vi "Autonomous Independent.vi"   [LabVIEW 2015]
doc: "This VI is called when autonomous begins, and will automatically be terminated when autonomous ends. You can carry out timed or sensor driven robot movement independently without needing to return to the caller."
uses:
  <vilib>/Rock Robotics/WPI/Solenoid/WPI_SolenoidValue.ctl
  <vilib>/Rock Robotics/WPI/Utilities/WPI_GetSetVariantRefNum.vi
  <vilib>/Rock Robotics/Network Tables/NT Read String.vi
  Robot Global Data.vi
  <vilib>/Rock Robotics/Network Tables/NT Write Number.vi
  <vilib>/Rock Robotics/WPI/Solenoid/Deprecated/WPI_SolenoidGetBool.vi
  <vilib>/Rock Robotics/WPI/Solenoid/WPI_SolenoidSetEnum.vi
  <vilib>/Rock Robotics/WPI/RobotDrive/WPI_RobotDriveArcadeDrive_Standard(NoSaturation).vi
  <vilib>/Rock Robotics/Network Tables/NT Write Numeric Array.vi
panel:
  # "Be sure to right-click and choose Data Operations>>Make Current Value default if you want to save the array values with the VI"
types:
  T1 = typedef "WPI_JoystickDevRef.ctl" = cluster{"Device":T2}
  T2 = typedef "WPI_JoystickDeviceEnum.ctl" = enum16{"USB 0", "USB 1", "USB 2", "USB 3", "USB 4", "USB 5"}
  T3 = typedef "WPI_SolenoidValue.ctl" = enum16{"Off", "On", "Forward", "Reverse"}
  T4 = typedef "WPI_RobotDriveDevRef.ctl" = cluster{"DevStatus":errorcluster, "Motors[]":T5[], "Square Inputs":bool, "Max Output":dbl}
  T5 = typedef "WPI_MotorControlDeviceRef.ctl" = cluster{"DeviceStatus":errorcluster, "Type":T6, "PWM":cluster{"PWM Channel":T7, "DeadBand":T8}, "CAN":cluster{"Device Number":u8, "Control Mode":T9, "Semaphore":T10, "Max Vout":dbl, "TalonSRX Control Mode":T11}, "Invert":bool}
  T6 = typedef "WPI_MotorControlType.ctl" = enum16{"PWM", "CAN", "CANTalonSRX"}
  T7 = typedef "FPGA_DIOPWMChannel.ctl" = enum8{"PWM 0", "PWM 1", "PWM 2", "PWM 3", "PWM 4", "PWM 5", "PWM 6", "PWM 7", "PWM 8", "PWM 9", "PWM MXP 0", "PWM MXP 1", "PWM MXP 2", "PWM MXP 3", "PWM MXP 4", "PWM MXP 5", "PWM MXP 6", "PWM MXP 7", "PWM MXP 8", "PWM MXP 9", "Invalid"}
  T8 = typedef "WPI_PWMDeadband.ctl" = cluster{"Name":string, "maxPositivePwm":i32, "minPositivePwm":i32, "centerPwm":i32, "maxNegativePwm":i32, "minNegativePwm":i32, "angularRange":u16}
  T9 = typedef "WPI_CANJaguar_ControlMode.ctl" = enum8{"Percent VBus", "Current", "Speed", "Position", "Voltage"}
  T10 = typedef "Semaphore RefNum" = refnum<k1>
  T11 = typedef "WPI_CANTalonSRX_APIControlMode.ctl" = enum8{"Percent VBus", "Speed", "Position", "Slave", "Unchanged / Invalid", "Voltage Compensation", "Current", "Motion Profile"}
  T12 = typedef "WPI_GyroDevRef.ctl" = cluster{"DevStatus":errorcluster, "Analog Channel":T13, "Offset":dbl, "Gain (VoltsPerDegree/Second)":dbl, "Gyro Type":enum16{"Analog", "XRS450"}, "Handle":i32, "SPI Bus":T14, "Device Found":bool, "Sample Rate":dbl, "Calibrate On Open":bool}
  T13 = typedef "FPGA_AIChannel.ctl" = enum8{"AI 0", "AI 1", "AI 2", "AI 3", "AI MXP 0", "AI MXP 1", "AI MXP 2", "AI MXP 3", "Invalid"}
  T14 = typedef "spi_bus.ctl" = enum16{"SPI On-Board, CS0", "SPI On-Board, CS1", "SPI On-Board, CS2", "SPI On-Board, CS3", "SPI MXP", "Invalid"}
  T15 = typedef "WPI_PotentiometerDevRef.ctl" = cluster{"DevStatus":errorcluster, "Analog Channel":T13, "Invert Output":bool}
  T16 = typedef "WPI_SolenoidDevRef.ctl" = cluster{"DevStatus":errorcluster, "Pneumatics Control Module":u8, "Forward Solenoid Channel":T17, "Reverse Solenoid Channel":T17}
  T17 = typedef "WPI_SolenoidChannel.ctl" = enum8{"Solenoid 0", "Solenoid 1", "Solenoid 2", "Solenoid 3", "Solenoid 4", "Solenoid 5", "Solenoid 6", "Solenoid 7", "Invalid"}
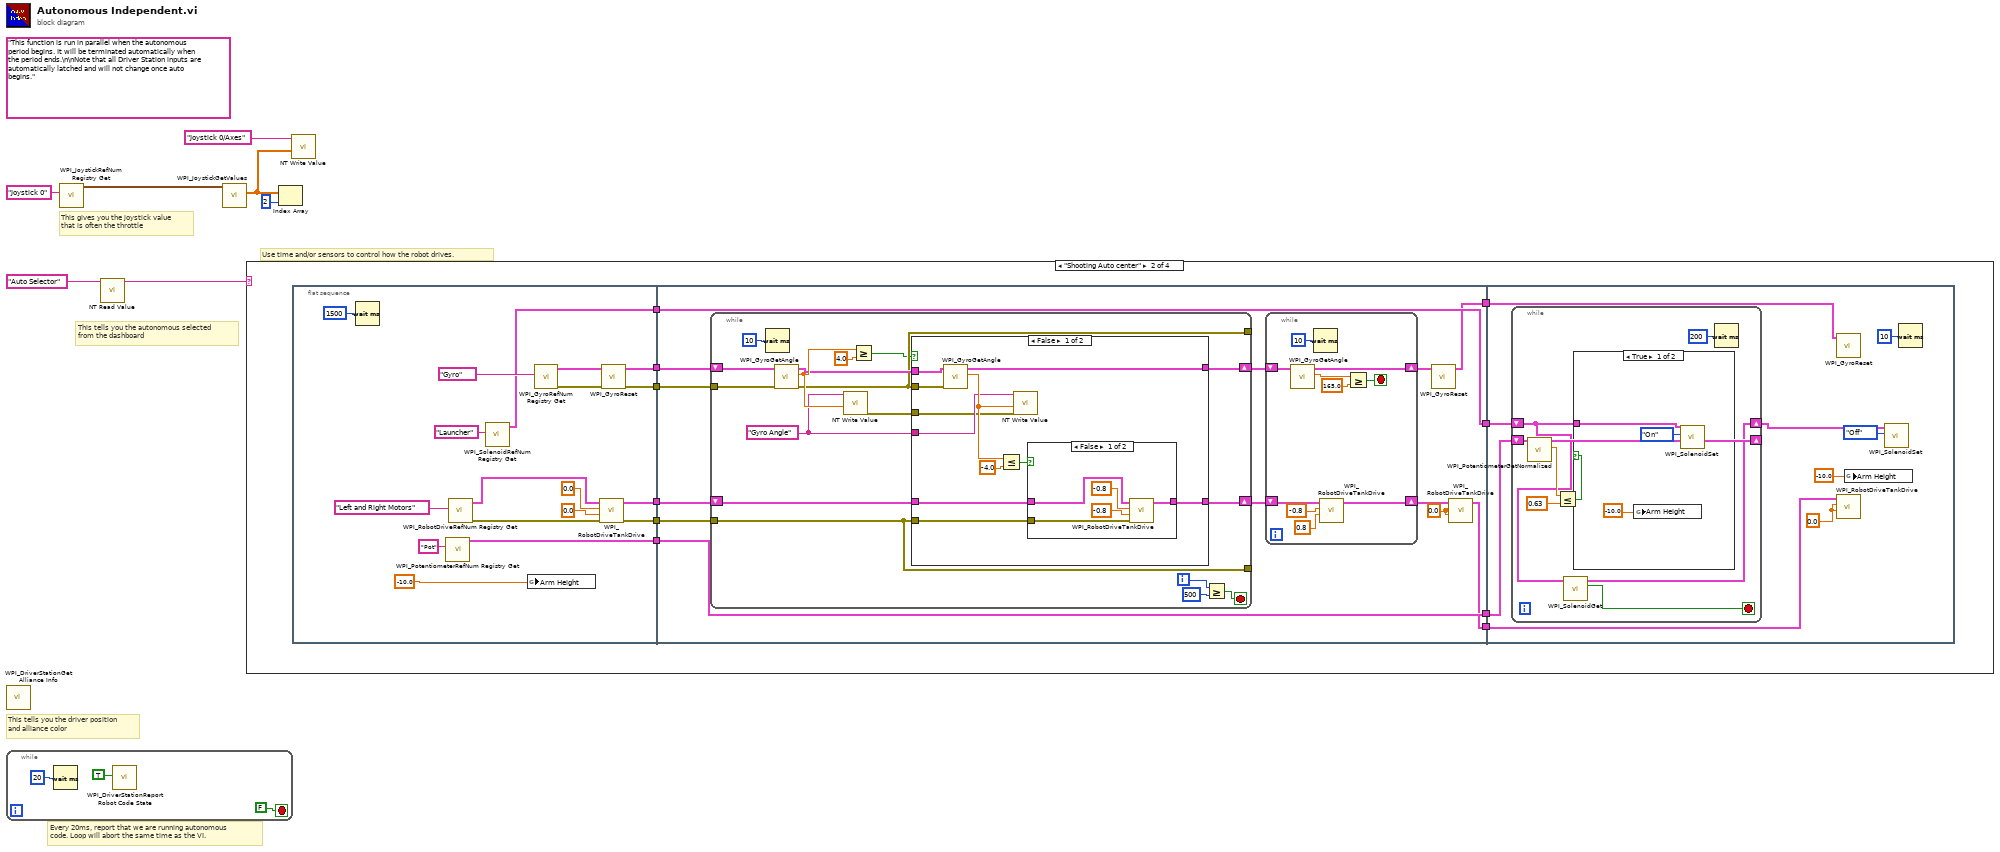
[diagram p0: block diagram]
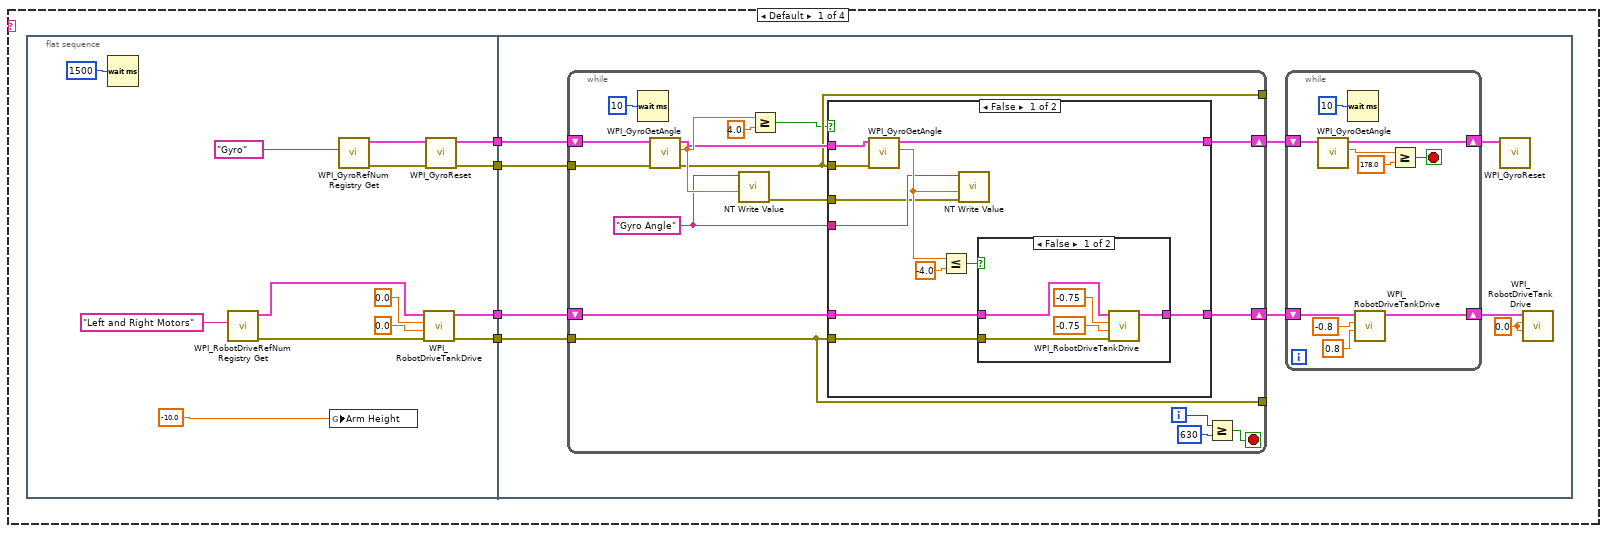
[diagram p2: hidden frame]
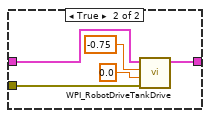
[diagram p3: hidden frame]
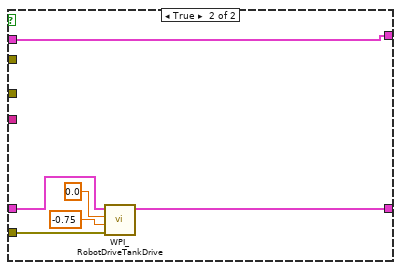
[diagram p4: hidden frame]
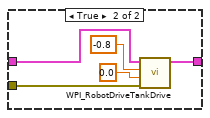
[diagram p5: hidden frame]
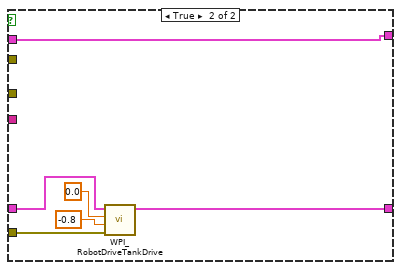
[diagram p6: hidden frame]
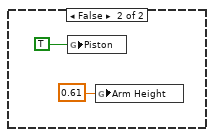
[diagram p7: hidden frame]
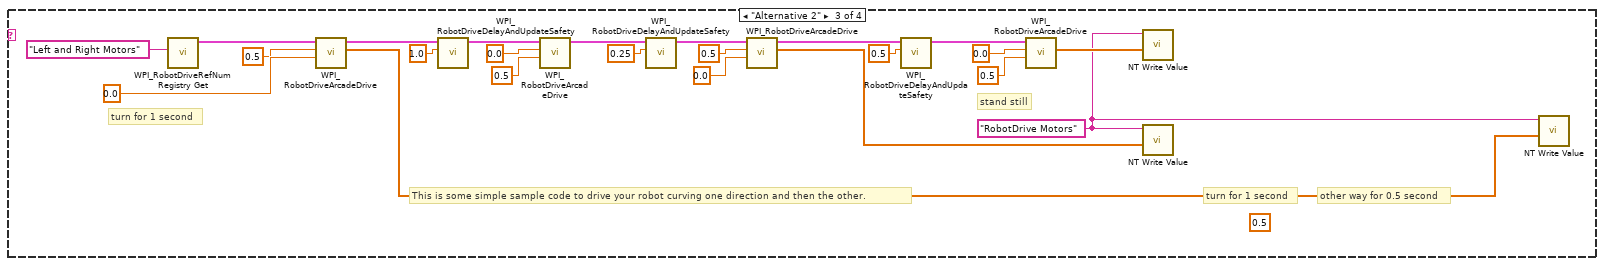
[diagram p8: hidden frame]
diagram:
  (unwired) "This function is run in parallel when the autonomous period begins. It will be terminated automatically when the period ends.\n\nNote that all Driver Station inputs are automatically latched and will not change once auto begins."
  # "This tells you the autonomous selected\nfrom the dashboard"
  # "Every 20ms, report that we are running autonomous\ncode. Loop will abort the same time as the VI."
  # "This gives you the joystick value\nthat is often the throttle"
  # "Use time and/or sensors to control how the robot drives."
  # "This tells you the driver position\nand alliance color"
  n1 = call <vilib>:"WPI_DriverStationGet Alliance Info.vi"() -> ()  [unwired: 12 out]
  n2 = while {
    stop <- FALSE stop-if-true
    n3 = Wait (ms)(milliseconds to wait=u32 20) -> ()  [unwired: 1 out]
    n4 = call <vilib>:"WPI_DriverStationReport Robot Code State.vi"("Autonomous"=TRUE) -> ()  [unwired: 10 in, 1 out]
  }
  n5 = call <vilib>:"WPI_JoystickRefNum Registry Get.vi"("refnum name"="Joystick 0") -> ("JoystickDevRef"=w6:T1)  [unwired: 1 in, 9 out]
  n6 = call-poly <vilib>:"NT Read Value.vi"("Name"="Auto Selector") -> ("String"=w3:string)  [unwired: 9 in, 1 out]
  n7 = call <vilib>:"WPI_JoystickGetValues.vi"("JoystickDevRef"=w6) -> ("Axes"=w2:dbl[])  [unwired: 6 in, 4 out]
  n8 = case shown="\"Shooting Auto center\"" w3 {
    frame Default {
      n9 = flat-sequence {
        tunnel: [w21] -> w14
        tunnel: [w20] -> w13
        tunnel: [w19] -> w12
        tunnel: [w18] -> w11
        tunnel: w14 -> [w37]
        tunnel: w13 -> [w36]
        tunnel: w12 -> [w35]
        tunnel: w11 -> [w34]
        frame #0 {
          n10 = Wait (ms)(milliseconds to wait=u32 1500) -> ()  [unwired: 1 out]
          n11 = call <vilib>:"WPI_RobotDriveRefNum Registry Get.vi"("refnum name"="Left and Right Motors") -> ("error out"=w24:errorcluster, "RobotDriveDevRef"=w25:T4)  [unwired: 9 in]
          n12 = global write "Robot Global Data.vi" "Arm Height"(-10.0) -> ()
          n13 = call <vilib>:"WPI_GyroRefNum Registry Get.vi"("refnum name"="Gyro") -> ("error out"=w27:errorcluster, "GyroDevRef"=w28:T12)  [unwired: 9 in]
          n14 = call <vilib>:"WPI_RobotDriveTankDrive.vi"("error in (no error)"=w24, "Right axis value"=0.0, "Left axis value"=0.0 ("Delay (s)"), "RobotDriveDevRef"=w25) -> ("error out"=w18:errorcluster, "RobotDriveDevRef"=w19:T4)  [unwired: 5 in, 1 out]
          n15 = call <vilib>:"WPI_GyroReset.vi"("error in"=w27, "GyroDevRef"=w28) -> ("error out"=w20:errorcluster, "GyroDevRef"=w21:T12)  [unwired: 8 in]
        }
        frame #1 {
          w30 = 0.0 ("Left axis value")
          n16 = while {
            tunnel: w36 -> [w61]
            tunnel: w34 -> [w56]
            tunnel: [w57] -> _
            tunnel: [w56] -> _
            shift-right: [w49] -> w33
            shift-left: w35 -> [w55]
            shift-right: [w48] -> w32
            shift-left: w37 -> [w64]
            i -> [w50]
            stop <- w62 stop-if-true
            w54 = "Gyro Angle" ("Name")
            n17 = Wait (ms)(milliseconds to wait=10) -> ()  [unwired: 1 out]
            n18 = call <vilib>:"WPI_GyroGetAngle.vi"("error in"=w61, "GyroDevRef"=w64) -> ("error out"=w57:errorcluster, "Angle"=w59:dbl, "GyroDevRef"=w58:T12)  [unwired: 5 in, 2 out]
            n19 = call-poly <vilib>:"NT Write Value.vi"("Numeric"=w59, "Name"=w54) -> ("error out"=w53:errorcluster)  [unwired: 9 in]
            n20 = Greater Or Equal?(x=w59, y=4.0) -> (x >= y?=w52:bool)
            n21 = case shown="False" w52 {
              tunnel: w56 -> [w71 w88]
              tunnel: w55 -> [w72 w89]
              tunnel: w58 -> [w75 w86]
              tunnel: w57 -> [w74 _]
              tunnel: w54 -> [w69 _]
              tunnel: w53 -> [w68 _]
              tunnel: [w66 w87] -> w49
              tunnel: [w65 w86] -> w48
              frame False {
                n22 = call <vilib>:"WPI_GyroGetAngle.vi"("error in"=w74, "GyroDevRef"=w75) -> ("Angle"=w70:dbl, "GyroDevRef"=w65:T12)  [unwired: 5 in, 3 out]
                n23 = Less Or Equal?(x=w70, y=-4.0) -> (x <= y?=w67:bool)
                n24 = call-poly <vilib>:"NT Write Value.vi"("error in"=w68, "Numeric"=w70, "Name"=w69) -> ()  [unwired: 8 in, 1 out]
                n25 = case shown="False" w67 {
                  tunnel: w72 -> [w80 w85]
                  tunnel: w71 -> [w79 w84]
                  tunnel: [w76 w81] -> w66
                  frame False {
                    n26 = call <vilib>:"WPI_RobotDriveTankDrive.vi"("error in (no error)"=w79, "Right axis value"=-0.75, "Left axis value"=-0.75, "RobotDriveDevRef"=w80) -> ("RobotDriveDevRef"=w76:T4)  [unwired: 5 in, 2 out]
                  }
                  frame True {
                    n27 = call <vilib>:"WPI_RobotDriveTankDrive.vi"("error in (no error)"=w84, "Right axis value"=0.0, "Left axis value"=-0.75, "RobotDriveDevRef"=w85) -> ("RobotDriveDevRef"=w81:T4)  [unwired: 5 in, 2 out]
                  }
                }
              }
              frame True {
                n28 = call <vilib>:"WPI_RobotDriveTankDrive.vi"("error in (no error)"=w88, "Right axis value"=-0.75, "Left axis value"=0.0, "RobotDriveDevRef"=w89) -> ("RobotDriveDevRef"=w87:T4)  [unwired: 5 in, 2 out]
              }
            }
            n29 = Greater Or Equal?(x=w50, y=u32 630) -> (x >= y?=w62:bool)
          }
          n30 = while {
            shift-right: [w39] -> w31
            shift-left: w32 -> [w46]
            shift-right: [w40] -> w29
            shift-left: w33 -> [w47]
            stop <- w41 stop-if-true
            n31 = call <vilib>:"WPI_GyroGetAngle.vi"("GyroDevRef"=w46) -> ("Angle"=w43:dbl, "GyroDevRef"=w39:T12)  [unwired: 6 in, 3 out]
            n32 = Wait (ms)(milliseconds to wait=u32 10) -> ()  [unwired: 1 out]
            n33 = call <vilib>:"WPI_RobotDriveTankDrive.vi"("Right axis value"=0.8, "Left axis value"=-0.8, "RobotDriveDevRef"=w47) -> ("RobotDriveDevRef"=w40:T4)  [unwired: 6 in, 2 out]
            n34 = Greater Or Equal?(x=w43, y=178.0) -> (x >= y?=w41:bool)
          }
          n35 = call <vilib>:"WPI_GyroReset.vi"("GyroDevRef"=w31) -> ()  [unwired: 9 in, 2 out]
          n36 = call <vilib>:"WPI_RobotDriveTankDrive.vi"("Right axis value"=w30, "Left axis value"=w30, "RobotDriveDevRef"=w29) -> ()  [unwired: 6 in, 3 out]
        }
      }
    }
    frame "Shooting Auto center" {
      n37 = flat-sequence {
        tunnel: [w112] -> w101
        tunnel: [w111] -> w100
        tunnel: [w110] -> w99
        tunnel: [w109] -> w98
        tunnel: [w103] -> w96
        tunnel: [w102] -> w94
        tunnel: w101 -> [w132]
        tunnel: w100 -> [w131]
        tunnel: w99 -> [w130]
        tunnel: w98 -> [w129]
        tunnel: [w123] -> w97
        tunnel: w96 -> [w123]
        tunnel: [w122] -> w95
        tunnel: w94 -> [w122]
        tunnel: [w121] -> w93
        tunnel: [w120] -> w92
        tunnel: w97 -> [w195]
        tunnel: w95 -> [w194]
        tunnel: w93 -> [w191]
        tunnel: w92 -> [w190]
        frame #0 {
          n38 = Wait (ms)(milliseconds to wait=u32 1500) -> ()  [unwired: 1 out]
          n39 = call <vilib>:"WPI_PotentiometerRefNum Registry Get.vi"("refnum name"="Pot") -> ("PotDevRef"=w103:T15)  [unwired: 9 in, 1 out]
          n40 = call <vilib>:"WPI_RobotDriveRefNum Registry Get.vi"("refnum name"="Left and Right Motors") -> ("error out"=w115:errorcluster, "RobotDriveDevRef"=w116:T4)  [unwired: 9 in]
          n41 = call <vilib>:"WPI_SolenoidRefNum Registry Get.vi"("refnum name"="Launcher") -> ("SolenoidDevRef"=w102:T16)  [unwired: 9 in, 1 out]
          n42 = global write "Robot Global Data.vi" "Arm Height"(-10.0) -> ()
          n43 = call <vilib>:"WPI_GyroRefNum Registry Get.vi"("refnum name"="Gyro") -> ("error out"=w118:errorcluster, "GyroDevRef"=w119:T12)  [unwired: 9 in]
          n44 = call <vilib>:"WPI_RobotDriveTankDrive.vi"("error in (no error)"=w115, "Right axis value"=0.0, "Left axis value"=0.0 ("Delay (s)"), "RobotDriveDevRef"=w116) -> ("error out"=w109:errorcluster, "RobotDriveDevRef"=w110:T4)  [unwired: 5 in, 1 out]
          n45 = call <vilib>:"WPI_GyroReset.vi"("error in"=w118, "GyroDevRef"=w119) -> ("error out"=w111:errorcluster, "GyroDevRef"=w112:T12)  [unwired: 8 in]
        }
        frame #1 {
          w125 = 0.0 ("Left axis value")
          n46 = while {
            tunnel: w131 -> [w156]
            tunnel: w129 -> [w151]
            tunnel: [w152] -> _
            tunnel: [w151] -> _
            shift-right: [w144] -> w128
            shift-left: w130 -> [w150]
            shift-right: [w143] -> w127
            shift-left: w132 -> [w159]
            i -> [w145]
            stop <- w157 stop-if-true
            w149 = "Gyro Angle" ("Name")
            n47 = Wait (ms)(milliseconds to wait=10) -> ()  [unwired: 1 out]
            n48 = call <vilib>:"WPI_GyroGetAngle.vi"("error in"=w156, "GyroDevRef"=w159) -> ("error out"=w152:errorcluster, "Angle"=w154:dbl, "GyroDevRef"=w153:T12)  [unwired: 5 in, 2 out]
            n49 = call-poly <vilib>:"NT Write Value.vi"("Numeric"=w154, "Name"=w149) -> ("error out"=w148:errorcluster)  [unwired: 9 in]
            n50 = Greater Or Equal?(x=w154, y=4.0) -> (x >= y?=w147:bool)
            n51 = case shown="False" w147 {
              tunnel: w151 -> [w166 w183]
              tunnel: w150 -> [w167 w184]
              tunnel: w153 -> [w170 w181]
              tunnel: w152 -> [w169 _]
              tunnel: w149 -> [w164 _]
              tunnel: w148 -> [w163 _]
              tunnel: [w161 w182] -> w144
              tunnel: [w160 w181] -> w143
              frame False {
                n52 = call <vilib>:"WPI_GyroGetAngle.vi"("error in"=w169, "GyroDevRef"=w170) -> ("Angle"=w165:dbl, "GyroDevRef"=w160:T12)  [unwired: 5 in, 3 out]
                n53 = Less Or Equal?(x=w165, y=-4.0) -> (x <= y?=w162:bool)
                n54 = call-poly <vilib>:"NT Write Value.vi"("error in"=w163, "Numeric"=w165, "Name"=w164) -> ()  [unwired: 8 in, 1 out]
                n55 = case shown="False" w162 {
                  tunnel: w167 -> [w175 w180]
                  tunnel: w166 -> [w174 w179]
                  tunnel: [w171 w176] -> w161
                  frame False {
                    n56 = call <vilib>:"WPI_RobotDriveTankDrive.vi"("error in (no error)"=w174, "Right axis value"=-0.8, "Left axis value"=-0.8, "RobotDriveDevRef"=w175) -> ("RobotDriveDevRef"=w171:T4)  [unwired: 5 in, 2 out]
                  }
                  frame True {
                    n57 = call <vilib>:"WPI_RobotDriveTankDrive.vi"("error in (no error)"=w179, "Right axis value"=0.0, "Left axis value"=-0.8, "RobotDriveDevRef"=w180) -> ("RobotDriveDevRef"=w176:T4)  [unwired: 5 in, 2 out]
                  }
                }
              }
              frame True {
                n58 = call <vilib>:"WPI_RobotDriveTankDrive.vi"("error in (no error)"=w183, "Right axis value"=-0.8, "Left axis value"=0.0, "RobotDriveDevRef"=w184) -> ("RobotDriveDevRef"=w182:T4)  [unwired: 5 in, 2 out]
              }
            }
            n59 = Greater Or Equal?(x=w145, y=u32 500) -> (x >= y?=w157:bool)
          }
          n60 = while {
            shift-right: [w134] -> w126
            shift-left: w127 -> [w141]
            shift-right: [w135] -> w124
            shift-left: w128 -> [w142]
            stop <- w136 stop-if-true
            n61 = call <vilib>:"WPI_GyroGetAngle.vi"("GyroDevRef"=w141) -> ("Angle"=w138:dbl, "GyroDevRef"=w134:T12)  [unwired: 6 in, 3 out]
            n62 = Wait (ms)(milliseconds to wait=u32 10) -> ()  [unwired: 1 out]
            n63 = call <vilib>:"WPI_RobotDriveTankDrive.vi"("Right axis value"=0.8, "Left axis value"=-0.8, "RobotDriveDevRef"=w142) -> ("RobotDriveDevRef"=w135:T4)  [unwired: 6 in, 2 out]
            n64 = Greater Or Equal?(x=w138, y=165.0) -> (x >= y?=w136:bool)
          }
          n65 = call <vilib>:"WPI_GyroReset.vi"("GyroDevRef"=w126) -> ("GyroDevRef"=w121:T12)  [unwired: 9 in, 1 out]
          n66 = call <vilib>:"WPI_RobotDriveTankDrive.vi"("Right axis value"=w125, "Left axis value"=w125, "RobotDriveDevRef"=w124) -> ("RobotDriveDevRef"=w120:T4)  [unwired: 6 in, 2 out]
        }
        frame #2 {
          w189 = 0.0
          n67 = while {
            shift-right: [w200] -> _
            shift-left: w195 -> [w201]
            shift-right: [w198] -> w193
            shift-left: w194 -> [w199]
            stop <- w197 stop-if-true
            n68 = call <vilib>:"WPI_PotentiometerGetNormalized.vi"("PotDevRef"=w201) -> ("Normalized Value"=w204:dbl, "PotDevRef"=w200:T15)  [unwired: 8 in, 1 out]
            n69 = Less Or Equal?(x=w204, y=0.63) -> (x <= y?=w202:bool)
            n70 = call-poly <vilib>:"WPI_SolenoidGet.vi"("SolenoidDevRef"=w199) -> ("Value"=w197:bool, "SolenoidDevRef"=w198:T16)  [unwired: 8 in, 1 out]
            n71 = case shown="True" w202 {
              tunnel: w199 -> [w205 _]
              frame True {
                n72 = global write "Robot Global Data.vi" "Arm Height"(-10.0) -> ()
                n73 = call-poly <vilib>:"WPI_SolenoidSet.vi"("Value"=WPI_SolenoidValue."On", "SolenoidDevRef"=w205) -> ()  [unwired: 8 in, 2 out]
              }
              frame False {
                n74 = global write "Robot Global Data.vi" "Piston"(TRUE ("Piston")) -> ()
                n75 = global write "Robot Global Data.vi" "Arm Height"(0.61) -> ()
              }
            }
            n76 = Wait (ms)(milliseconds to wait=u32 200) -> ()  [unwired: 1 out]
          }
          n77 = call <vilib>:"WPI_GyroReset.vi"("GyroDevRef"=w191) -> ()  [unwired: 9 in, 2 out]
          n78 = call <vilib>:"WPI_RobotDriveTankDrive.vi"("Right axis value"=w189, "Left axis value"=w189, "RobotDriveDevRef"=w190) -> ()  [unwired: 6 in, 3 out]
          n79 = global write "Robot Global Data.vi" "Arm Height"(-10.0) -> ()
          n80 = call-poly <vilib>:"WPI_SolenoidSet.vi"("Value"=WPI_SolenoidValue."Off", "SolenoidDevRef"=w193) -> ()  [unwired: 8 in, 2 out]
          n81 = Wait (ms)(milliseconds to wait=u32 10) -> ()  [unwired: 1 out]
        }
      }
    }
    frame "Alternative 2" {
      (unwired) 0.5 ("X axis value")
      w220 = "RobotDrive Motors" ("Name")
      # "turn for 1 second"
      # "This is some simple sample code to drive your robot curving one direction and then the other."
      # "stand still"
      # "other way for 0.5 second"
      # "turn for 1 second"
      n82 = call <vilib>:"WPI_RobotDriveRefNum Registry Get.vi"("refnum name"="Left and Right Motors") -> ("RobotDriveDevRef"=w232:T4)  [unwired: 1 in, 9 out]
      n83 = call-poly <vilib>:"WPI_RobotDriveArcadeDrive.vi"("Y axis value"=0.0 ("X axis value"), "X axis value"=0.5, "RobotDriveDevRef"=w232) -> ("Motor Values"=w219:dbl[], "RobotDriveDevRef"=w226:T4)  [unwired: 1 in, 6 out]
      n84 = call <vilib>:"WPI_RobotDriveDelayAndUpdateSafety.vi"("Delay (s)"=1.0, "RobotDriveDevRef"=w226) -> ("RobotDriveDevRef 2"=w217:T4)  [unwired: 8 in, 1 out]
      n85 = call-poly <vilib>:"WPI_RobotDriveArcadeDrive.vi"("Y axis value"=0.5 ("X axis value"), "X axis value"=0.0, "RobotDriveDevRef"=w217) -> ("RobotDriveDevRef"=w214:T4)  [unwired: 1 in, 7 out]
      n86 = call <vilib>:"WPI_RobotDriveDelayAndUpdateSafety.vi"("Delay (s)"=0.25, "RobotDriveDevRef"=w214) -> ("RobotDriveDevRef 2"=w213:T4)  [unwired: 8 in, 1 out]
      n87 = call-poly <vilib>:"WPI_RobotDriveArcadeDrive.vi"("Y axis value"=0.0 ("X axis value"), "X axis value"=0.5, "RobotDriveDevRef"=w213) -> ("Motor Values"=w221:dbl[], "RobotDriveDevRef"=w227:T4)  [unwired: 1 in, 6 out]
      n88 = call <vilib>:"WPI_RobotDriveDelayAndUpdateSafety.vi"("Delay (s)"=0.5, "RobotDriveDevRef"=w227) -> ("RobotDriveDevRef 2"=w228:T4)  [unwired: 8 in, 1 out]
      n89 = call-poly <vilib>:"WPI_RobotDriveArcadeDrive.vi"("Y axis value"=0.5 ("X axis value"), "X axis value"=0.0, "RobotDriveDevRef"=w228) -> ("Motor Values"=w222:dbl[])  [unwired: 1 in, 7 out]
      n90 = call-poly <vilib>:"NT Write Value.vi"("Numeric Array"=w222, "Name"=w220) -> ()  [unwired: 9 in, 1 out]
      n91 = call-poly <vilib>:"NT Write Value.vi"("Numeric Array"=w221, "Name"=w220) -> ()  [unwired: 9 in, 1 out]
      n92 = call-poly <vilib>:"NT Write Value.vi"("Numeric Array"=w219, "Name"=w220) -> ()  [unwired: 9 in, 1 out]
    }
    frame "Your Turn" {
    }
  }
  n93 = Index Array(array=w2, index=2) -> ()  [unwired: 1 out]
  n94 = call-poly <vilib>:"NT Write Value.vi"("Numeric Array"=w2, "Name"="Joystick 0/Axes") -> ()  [unwired: 9 in, 1 out]
